vi "LAC Cmd119R_Meas luminance.vi"(7 "timeout(ms)":u32=500, 8 "error in":errorcluster, 11 "VISA name in":refnum<visa-resource-name>) -> (0 "error out":errorcluster, 1 "Luminance read":string, 3 "VISA name out":refnum<visa-resource-name>)   [LabVIEW 2018]
panel:
  # "readout item\n\n*1: Measurement luminance value \n      (0 to 4095)"
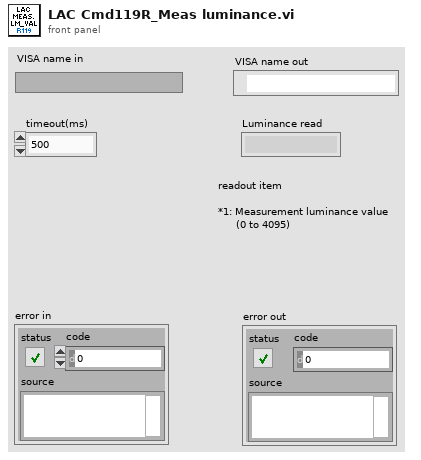
[diagram p1: front panel]
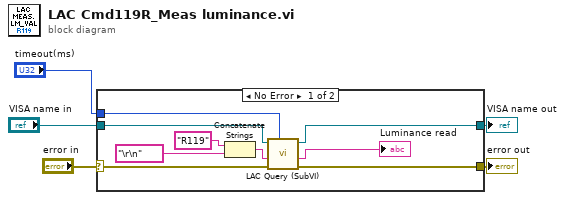
[diagram p0: block diagram]
diagram:
  n1 = case shown="No Error" "error in" {
    selector: "error in" -> [w10 w16]
    tunnel: "VISA name in" -> [w12 w15]
    tunnel: [w14 w15] -> w4
    tunnel: [w13 w16] -> w3
    tunnel: "timeout(ms)" -> [w11 _]
    frame No Error {
      n2 = Concatenate Strings("R119" ("string"), "\r\n" ("write buffer")) -> (w8:string)
      n3 = call "LAC Query (SubVI).vi"("timeout(ms)"=w11, "error in"=w10, "Command"=w8, "VISA name in"=w12) -> ("error out"=w13:errorcluster, "read buffer"=→"Luminance read":string, "VISA name out"=w14:refnum<visa-resource-name>)  [unwired: 5 in]
    }
    frame Error {
    }
  }
  "VISA name out" <- w4
  "error out" <- w3
